vi "Generate Unique Header.vi"(8 "error in":errorcluster, 11 "ePAS Cell Data in":refnum<class "ePAS Cell Data.lvclass">) -> (0 "error out":errorcluster, 2 "Header":string[](array[string]), 3 "ePAS Cell Data out":refnum<class "ePAS Cell Data.lvclass">)   [LabVIEW 2014, in "ePAS Library.lvlib" / "ePAS Cell Data.lvclass"]
uses:
  ePAS Cell Data.lvclass
  reusable/Data/Data.lvclass/Data.ctl
  reusable/Data/Read Data ID.vi
  reusable/PAS/Data/Cell/PAS Cell Data.lvclass
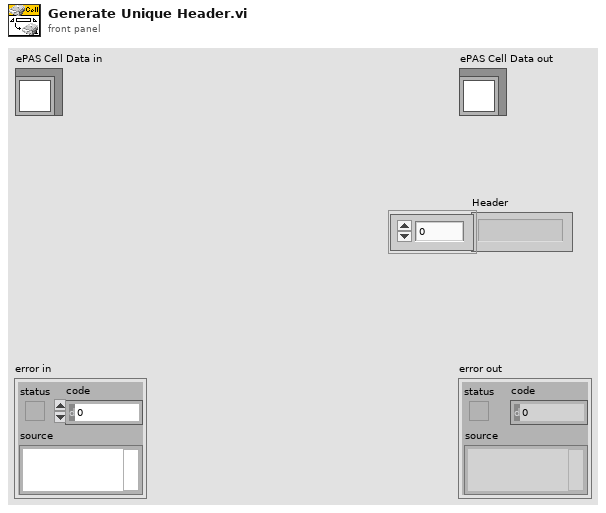
[diagram p1: front panel]
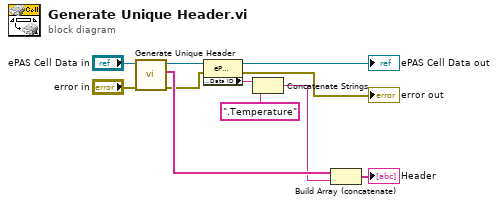
[diagram p0: block diagram]
diagram:
  n1 = call-parent "Generate Unique Header.vi"("error in"="error in", "PAS Cell Data in"="ePAS Cell Data in") -> ("error out"=w5:errorcluster, "Header"=w9:string[], "PAS Cell Data out"=w7:refnum<class "ePAS Cell Data.lvclass">)  [unwired: 7 in]
  n2 = property class="ePAS Cell"(reference=w7, error in=w5) -> (reference out=→"ePAS Cell Data out":refnum<class "ePAS Cell Data.lvclass">, error out=→"error out":errorcluster, "Accessors:Data ID"=w3:string)
  n3 = Concatenate Strings(w3, ".Temperature") -> (w1:string)
  n4 = Build Array (concatenate)(w9, w1) -> (→"Header":string[])
